vi "HTTP-GetAuth.vi"(8 "error in (no error)":errorcluster, 10 "Password":string, 11 "ByteGSWebAPI-V0 in":refnum<class "ByteGSWebAPI-V0.lvclass">) -> (0 "error out":errorcluster, 3 "ByteGSWebAPI-V0 out":refnum<class "ByteGSWebAPI-V0.lvclass">)   [LabVIEW 2019, in "ByteGSWebAPI.lvlib" / "ByteGSWebAPI-V0.lvclass"]
doc: "Richiede al server il token di autorizzazione.\nPassword necessaria per la richiesta."
uses:
  ByteGSWebAPI-V0.lvclass
  Connect/ConnectReply.ctl
  ByteGSWebAPI-V0.lvclass/ByteGSWebAPI-V0.ctl
  139c0e9b-ca58-4deb-b816-c04ecae34641.vi
  <vilib>/httpClient/POSTBuffer.vi
  <vilib>/JDP Science/JSONtext/JSON text to Variant.vi
  <vilib>/JDP Science/JSONtext/LVClass Serializer/JSONtext LVClass Serializer.lvclass
  <vilib>/httpClient/LabVIEWHTTPClient.lvlib
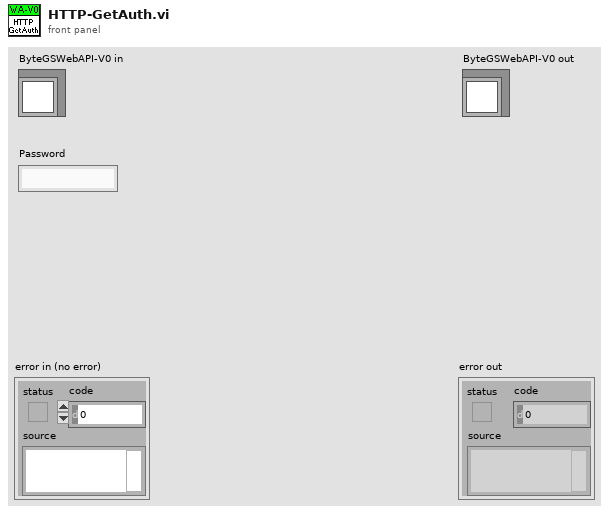
[diagram p1: front panel]
types:
  T1 = typedef "ByteGSWebAPI.lvlib/ByteGSWebAPI-V0.lvclass/ConnectReply.ctl" = cluster{"token":string}
  T2 = typedef "LabVIEWHTTPClient.lvlib/ClientHandle.ctl" = refnum<k1>
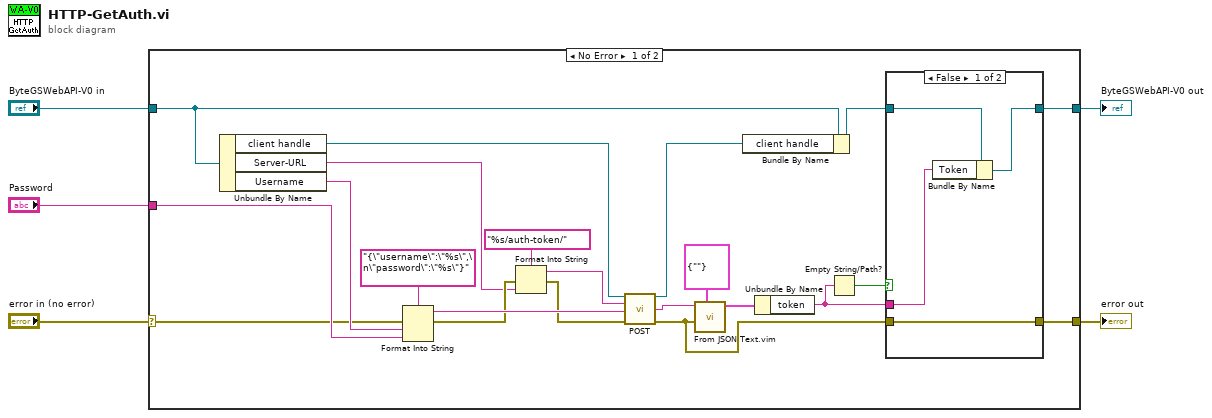
[diagram p0: block diagram]
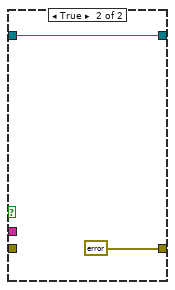
[diagram p2: hidden frame]
diagram:
  n1 = case shown="No Error" "error in (no error)" {
    selector: "error in (no error)" -> [w21 w35]
    tunnel: [w11 w35] -> w4
    tunnel: [w12 w34] -> w2
    tunnel: "ByteGSWebAPI-V0 in" -> [w13 w34]
    tunnel: "Password" -> [w22 _]
    frame No Error {
      n2 = Unbundle By Name(w13) -> ("client handle"=w9:T2, "Server-URL"=w8:string, "Username"=w23:string)
      n3 = Format Into String(format string="{\"username\":\"%s\",\n\"password\":\"%s\"}" ("buffer"), error in=w21, w23, w22) -> (resulting string=w24:string, error out=w20:errorcluster)  [unwired: 1 in]
      n4 = Format Into String(format string="%s/auth-token/" ("url"), error in=w20, w8) -> (resulting string=w26:string, error out=w19:errorcluster)  [unwired: 1 in]
      n5 = call-poly <vilib>:"POST.vi"("client handle"=w9, "url"=w26, "buffer"=w24, "error in (no error)"=w19) -> ("client handle out"=w6:T2, "body"=w17:string, "error out"=w10:errorcluster)  [unwired: 8 in, 1 out]
      n6 = call "From JSON Text.vim"("Data Type and Default Value"=T1 {"token"=""} ("ConnectReply"), "error in (no error)"=w10, "JSON"=w17) -> ("Data out"=w16:T1)  [unwired: 7 in, 1 out]
      n7 = Bundle By Name(cluster=w13, "client handle"=w6) -> (w7:refnum<class "ByteGSWebAPI-V0.lvclass">)
      n8 = Unbundle By Name(w16) -> ("token"=w14:string)
      n9 = Empty String/Path?(string/path=w14) -> (empty?=w15:bool)
      n10 = case shown="False" w15 {
        tunnel: w14 -> [w30 _]
        tunnel: w7 -> [w31 w33]
        tunnel: [w29 w33] -> w12
        tunnel: [w28 errorcluster {"status"=TRUE, "code"=0, "source"="Empty Token"} ("error in (no error)")] -> w11
        tunnel: w10 -> [w28 _]
        frame False {
          n11 = Bundle By Name(cluster=w31, "Token"=w30) -> (w29:refnum<class "ByteGSWebAPI-V0.lvclass">)
        }
        frame True {
        }
      }
    }
    frame Error {
    }
  }
  "error out" <- w4
  "ByteGSWebAPI-V0 out" <- w2
